vi "Test JL Display.vi"(0 "Expected LEDs":T7={"SSD"="", "Cycle Selection"=enum."Cycle 0", "Bar Selection"=enum."Bar 1", "Temp Setting"=enum."High", "Dryness Level"=enum."Damp", "Time Setting"=enum."Default Time 1", "Dryer Status"=enum."Status 1", "Start/Pause"=FALSE, "Pause"=FALSE, "Control Lock"=FALSE, "Sensing"=FALSE, "Clean Filter"=FALSE, "My Cycle"=FALSE, "Delay Dry"=FALSE, "Volume"=FALSE, "Damp Alert"=FALSE, "Ext Tumble"=FALSE, "Decrement"=FALSE, "Increment"=FALSE, "eDry"=FALSE, "Extra Status"=FALSE}, 5 "Care?":T8, 7 "Actual LEDs":T7={"SSD"="", "Cycle Selection"=enum."Cycle 0", "Bar Selection"=enum."Bar 1", "Temp Setting"=enum."High", "Dryness Level"=enum."Damp", "Time Setting"=enum."Default Time 1", "Dryer Status"=enum."Status 1", "Start/Pause"=FALSE, "Pause"=FALSE, "Control Lock"=FALSE, "Sensing"=FALSE, "Clean Filter"=FALSE, "My Cycle"=FALSE, "Delay Dry"=FALSE, "Volume"=FALSE, "Damp Alert"=FALSE, "Ext Tumble"=FALSE, "Decrement"=FALSE, "Increment"=FALSE, "eDry"=FALSE, "Extra Status"=FALSE}, 11 "error in":errorcluster) -> (4 "Pass/Fail?":bool, 6 "Report Text":string, 15 "error out":errorcluster)   [LabVIEW 2016]
uses:
  type defs/JL Display.ctl
  type defs/Cycle Selection Enum.ctl
  type defs/Bar Enum.ctl
  type defs/Temp Setting Enum.ctl
  type defs/Dryness Enum.ctl
  type defs/Time Enum.ctl
  type defs/Status Enum.ctl
  type defs/JL Display Care.ctl
panel:
  in  "Bar Selection":T1
  in  "Time Setting":T2=enum."Default Time 1"
  in  "Temp Setting":T3=enum."No Heat"
  in  "Dryer Status":T4
  in  "Dryness Level":T5=enum."Damp"
  in  "Cycle Selection":T6
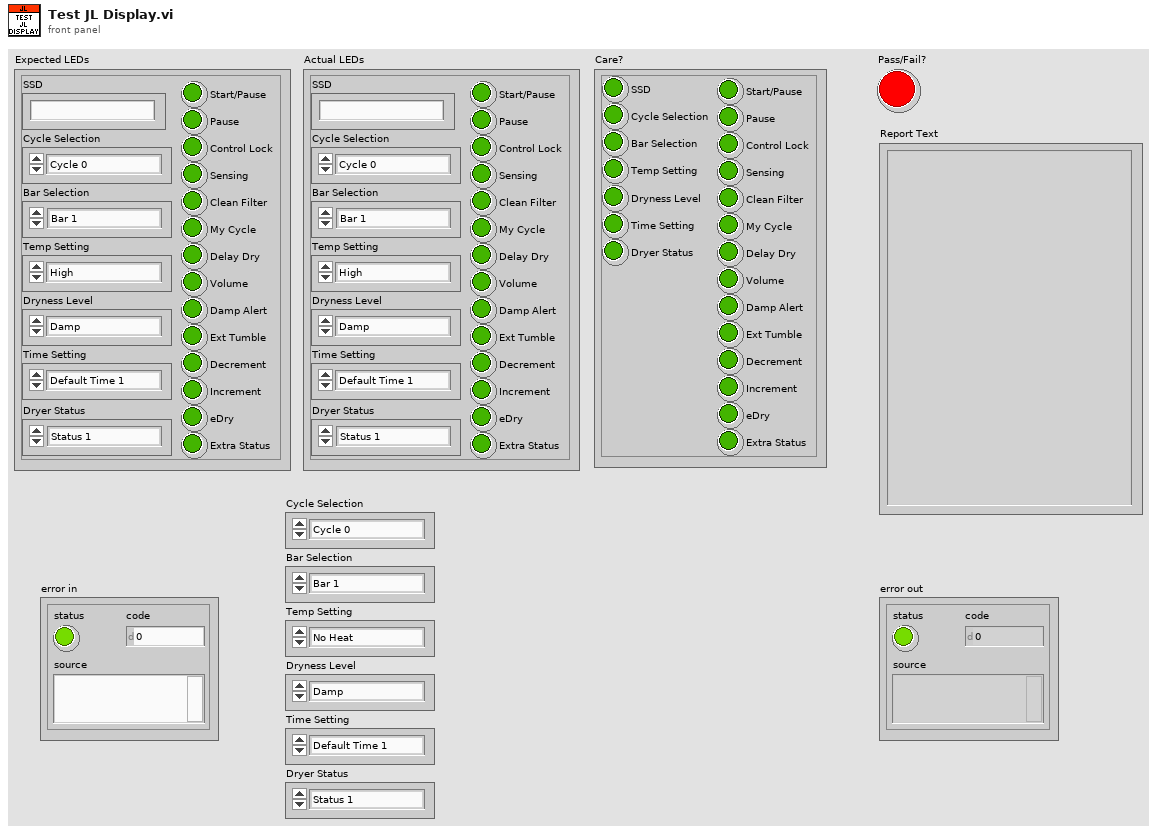
[diagram p1: front panel]
types:
  T1 = typedef "Bar Enum.ctl" = enum16{"Bar 1", "Bar 2", "Bar 3", "Bar 4", "Bar 5", "Off", "*Incorrect*"}
  T2 = typedef "Time Enum.ctl" = enum16{"Off", "Default Time 1", "Default Time 2", "Default Time 3", "Default Time 4", "Default Time 5", "*Incorrect*"}
  T3 = typedef "Temp Setting Enum.ctl" = enum16{"Off", "No Heat", "Extra Low", "Low", "Medium", "High", "*Incorrect*"}
  T4 = typedef "Status Enum.ctl" = enum16{"Status 1", "Status 2", "Status 3", "Status 4", "Status 5", "Status 6", "Off", "*Incorrect*"}
  T5 = typedef "Dryness Enum.ctl" = enum16{"Off", "Damp", "Less Dry", "Dry", "More Dry", "Extra Dry", "*Incorrect*"}
  T6 = typedef "Cycle Selection Enum.ctl" = enum16{"Cycle 0", "Cycle 1", "Cycle 2", "Cycle 3", "Cycle 4", "Cycle 5", "Cycle 6", "Cycle 7", "Cycle 8", "Cycle 9", "Cycle 10", "Cycle 11", "Cycle 12", "Cycle 13", "Off", "*Invalid"}
  T7 = typedef "JL Display.ctl" = cluster{"SSD":string, "Cycle Selection":T6, "Bar Selection":T1, "Temp Setting":T3, "Dryness Level":T5, "Time Setting":T2, "Dryer Status":T4, "Start/Pause":bool, "Pause":bool, "Control Lock":bool, "Sensing":bool, "Clean Filter":bool, "My Cycle":bool, "Delay Dry":bool, "Volume":bool, "Damp Alert":bool, "Ext Tumble":bool, "Decrement":bool, "Increment":bool, "eDry":bool, "Extra Status":bool}
  T8 = typedef "JL Display Care.ctl" = cluster{"SSD":bool, "Cycle Selection":bool, "Bar Selection":bool, "Temp Setting":bool, "Dryness Level":bool, "Time Setting":bool, "Dryer Status":bool, "Start/Pause":bool, "Pause":bool, "Control Lock":bool, "Sensing":bool, "Clean Filter":bool, "My Cycle":bool, "Delay Dry":bool, "Volume":bool, "Damp Alert":bool, "Ext Tumble":bool, "Decrement":bool, "Increment":bool, "eDry":bool, "Extra Status":bool}
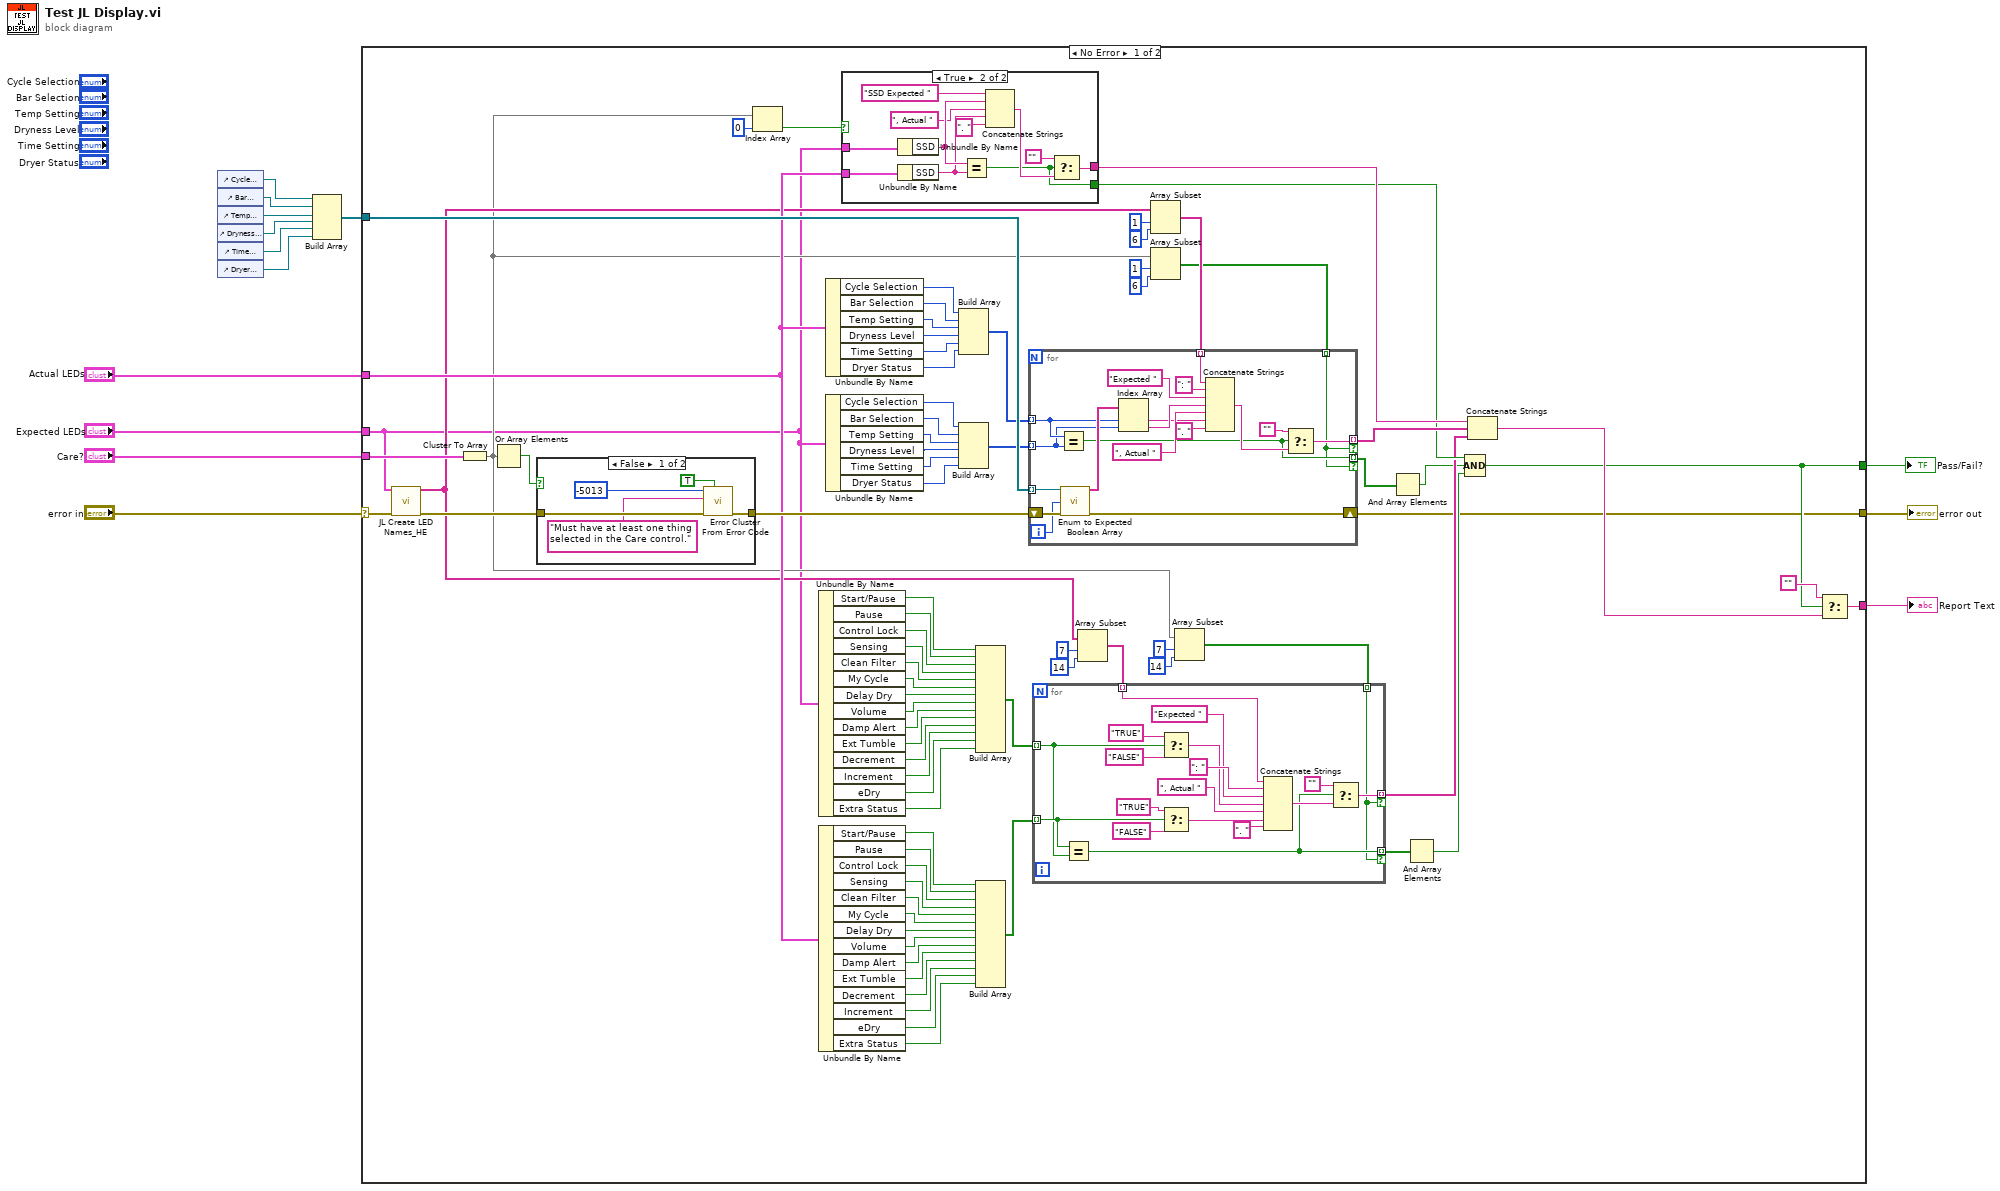
[diagram p0: block diagram]
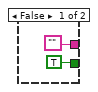
[diagram p2: hidden frame]
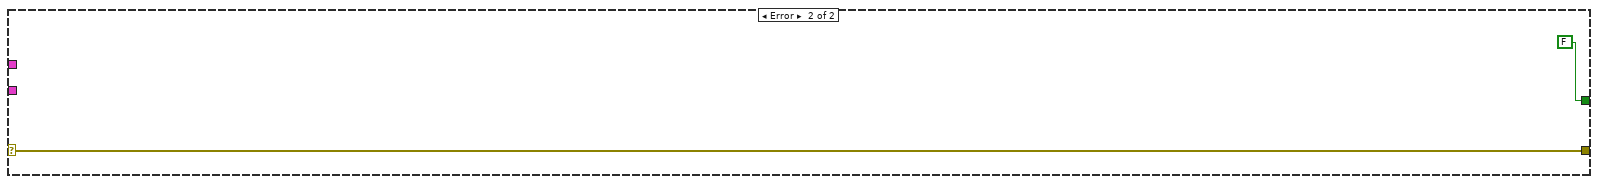
[diagram p4: hidden frame]
diagram:
  n1 = control-ref of="Cycle Selection"() -> (w6:refnum<vi>)
  n2 = control-ref of="Bar Selection"() -> (w5:refnum<vi>)
  n3 = control-ref of="Temp Setting"() -> (w4:refnum<vi>)
  n4 = control-ref of="Dryness Level"() -> (w3:refnum<vi>)
  n5 = control-ref of="Time Setting"() -> (w2:refnum<vi>)
  n6 = control-ref of="Dryer Status"() -> (w1:refnum<vi>)
  n7 = Build Array(w6, w5, w4, w3, w2, w1) -> (w7:refnum<vi>[])
  n8 = case shown="No Error" "error in" {
    selector: "error in" -> [w93 w153]
    tunnel: [w27 w153] -> w14
    tunnel: [w94 _] -> w13
    tunnel: "Care?" -> [w91 _]
    tunnel: "Expected LEDs" -> [w17 _]
    tunnel: "Actual LEDs" -> [w46 _]
    tunnel: [w28 FALSE] -> w8
    tunnel: w7 -> [w85 _]
    frame No Error {
      n9 = call "JL Create LED Names_HE.vi"("Expected LEDs"=w17, "Error In"=w93) -> ("Array of LED Names"=w37:string[], "Error Out"=w90:errorcluster)  [unwired: 12 in]
      n10 = Cluster To Array(cluster=w91) -> (array=w18:bool[])
      n11 = Or Array Elements(Boolean array=w18) -> (logical OR=w92:bool)
      n12 = case shown="False" w92 {
        tunnel: w90 -> [w150 w151]
        tunnel: [w149 w151] -> w74
        frame False {
          n13 = call <vilib>:"Error Cluster From Error Code.vi"("show call chain? (False)"=TRUE, "error in (no error)"=w150, "error message (\"\")"="Must have at least one thing selected in the Care control." ("error message (\"\")"), "error code (0)"=-5013) -> ("error out"=w149:errorcluster)  [unwired: 5 in]
        }
        frame True {
        }
      }
      n14 = Index Array(array=w18, index=0) -> (element=w43:bool)
      n15 = Unbundle By Name(w17) -> ("Start/Pause"=w60:bool, "Pause"=w59:bool, "Control Lock"=w58:bool, "Sensing"=w57:bool, "Clean Filter"=w56:bool, "My Cycle"=w55:bool, "Delay Dry"=w54:bool, "Volume"=w53:bool, "Damp Alert"=w52:bool, "Ext Tumble"=w51:bool, "Decrement"=w50:bool, "Increment"=w49:bool, "eDry"=w22:bool, "Extra Status"=w21:bool)
      n16 = Unbundle By Name(w46) -> ("Start/Pause"=w72:bool, "Pause"=w71:bool, "Control Lock"=w70:bool, "Sensing"=w69:bool, "Clean Filter"=w68:bool, "My Cycle"=w67:bool, "Delay Dry"=w66:bool, "Volume"=w65:bool, "Damp Alert"=w64:bool, "Ext Tumble"=w63:bool, "Decrement"=w62:bool, "Increment"=w61:bool, "eDry"=w20:bool, "Extra Status"=w19:bool)
      n17 = Unbundle By Name(w46) -> ("Cycle Selection"=w25:T6, "Bar Selection"=w26:T1, "Temp Setting"=w89:T3, "Dryness Level"=w88:T5, "Time Setting"=w87:T2, "Dryer Status"=w86:T4)
      n18 = Unbundle By Name(w17) -> ("Cycle Selection"=w23:T6, "Bar Selection"=w24:T1, "Temp Setting"=w77:T3, "Dryness Level"=w78:T5, "Time Setting"=w79:T2, "Dryer Status"=w80:T4)
      n19 = case shown="True" w43 {
        tunnel: ["" w119] -> w73
        tunnel: w46 -> [_ w118]
        tunnel: w17 -> [_ w117]
        tunnel: [TRUE w116] -> w45
        frame False {
        }
        frame True {
          n20 = Unbundle By Name(w117) -> ("SSD"=w124:string)
          n21 = Unbundle By Name(w118) -> ("SSD"=w122:string)
          n22 = Equal?(x=w124, y=w122) -> (x = y?=w116:bool)
          n23 = Concatenate Strings("SSD Expected " ("string"), w124, ", Actual " ("string"), w122, ". " ("string")) -> (w120:string)
          n24 = Select(t="", s=w116, f=w120) -> (s? t:f=w119:string)
        }
      }
      n25 = Build Array(w25, w26, w89, w88, w87, w86) -> (w84:u16[])
      n26 = Build Array(w23, w24, w77, w78, w79, w80) -> (w76:u16[])
      n27 = Build Array(w60, w59, w58, w57, w56, w55, w54, w53, w52, w51, w50, w49, w22, w21) -> (w41:bool[])
      n28 = Build Array(w72, w71, w70, w69, w68, w67, w66, w65, w64, w63, w62, w61, w20, w19) -> (w42:bool[])
      n29 = Array Subset(array=w37, index=7, length=14) -> (w38:string[])
      n30 = Array Subset(array=w37, index=1, length=6) -> (w81:string[])
      n31 = Array Subset(array=w18, index=1, length=6) -> (w15:bool[])
      n32 = for {
        tunnel: w85 -> [w128] mode=indexing
        shift-right: [w144] -> w27
        shift-left: w74 -> [w145]
        tunnel: w84 -> [w141] mode=indexing
        tunnel: w76 -> [w140] mode=indexing
        tunnel: w81 -> [w139] mode=indexing
        tunnel: [w131] -> w75 mode=indexing if=w129
        tunnel: [w130] -> w31 mode=indexing if=w129
        tunnel: w15 -> [w129] mode=indexing
        i -> [w127]
        n33 = Equal?(x=w141, y=w140) -> (x = y?=w130:bool)
        n34 = call "Enum to Expected Boolean Array.vi"("reference"=w128, "index"=w127, "error in (no error)"=w145) -> ("Enum Names"=w142:string[], "error out"=w144:errorcluster)  [unwired: 10 in, 1 out]
        n35 = Index Array(array=w142, index #1=w141, index #2=w140) -> (element #1=w134:string, element #2=w136:string)
        n36 = Concatenate Strings(w139, ": " ("string"), "Expected " ("string"), w136, ", Actual " ("string"), w134, ". " ("string")) -> (w132:string)
        n37 = Select(t="", s=w130, f=w132) -> (s? t:f=w131:string)
      }
      n38 = Array Subset(array=w18, index=7, length=14) -> (w16:bool[])
      n39 = for {
        tunnel: w42 -> [w104] mode=indexing
        tunnel: w41 -> [w98] mode=indexing
        tunnel: [w107] -> w34 mode=indexing if=w105
        tunnel: [w106] -> w30 mode=indexing if=w105
        tunnel: w16 -> [w105] mode=indexing
        tunnel: w38 -> [w96] mode=indexing
        n40 = Equal?(x=w104, y=w98) -> (x = y?=w106:bool)
        n41 = Select(t="TRUE" ("string"), s=w98, f="FALSE" ("string")) -> (s? t:f=w97:string)
        n42 = Select(t="TRUE" ("string"), s=w104, f="FALSE" ("string")) -> (s? t:f=w101:string)
        n43 = Concatenate Strings(w96, ": " ("string"), "Expected " ("string"), w97, ", Actual " ("string"), w101, ". " ("string")) -> (w108:string)
        n44 = Select(t="", s=w106, f=w108) -> (s? t:f=w107:string)
      }
      n45 = And Array Elements(Boolean array=w31) -> (logical AND=w32:bool)
      n46 = And Array Elements(Boolean array=w30) -> (logical AND=w29:bool)
      n47 = Compound Arithmetic op=AND(w45, w32, w29) -> (w28:bool)
      n48 = Concatenate Strings(w73, w75, w34) -> (w33:string)
      n49 = Select(t="", s=w28, f=w33) -> (s? t:f=w94:string)
    }
    frame Error {
    }
  }
  "error out" <- w14
  "Pass/Fail?" <- w8
  "Report Text" <- w13
